vi "MultiAxisPositioningWithTime.vi"(0 "connection ID":refnum<k5>, 1 "set1":bool=TRUE, 2 "set2":bool=TRUE, 3 "set3":bool=TRUE, 4 "target1":i32, 5 "error":errorcluster, 6 "target2":i32, 7 "target3":i32) -> (14 "connection ID out":refnum<k5>, 15 "Output parameters":T1, 19 "error out":errorcluster)   [LabVIEW 2016, in "amc_api.lvlib"]
doc: "In addition to \"MultiAxisPositioning\", this function returns a timestamp to the current position of each axis."
uses:
  amc_api.lvlib
panel:
  out "jsonRespIn":string
  out "JSON-response":string="{\"jsonrpc\":\"2.0\",\"method\":\"\",\"params\":[5,1.245,true,\"name\"],\"id\":\"1\"}"
  out "JSON request":string
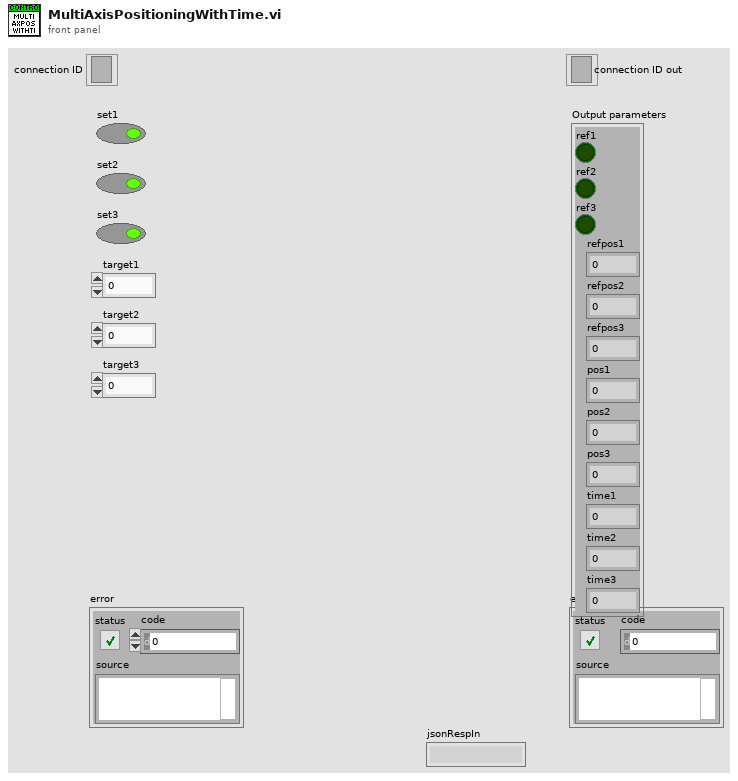
[diagram p1: front panel]
types:
  T1 = cluster{"ref1":bool, "ref2":bool, "ref3":bool, "refpos1":i32, "refpos2":i32, "refpos3":i32, "pos1":i32, "pos2":i32, "pos3":i32, "time1":dbl, "time2":dbl, "time3":dbl}
  T2 = cluster{"jsonrpc":string, "method":string, "params":string[], "id":string, "api":i32, "pid":string}
  T3 = enum16{"Standard", "Buffered", "CRLF", "Immediate"}
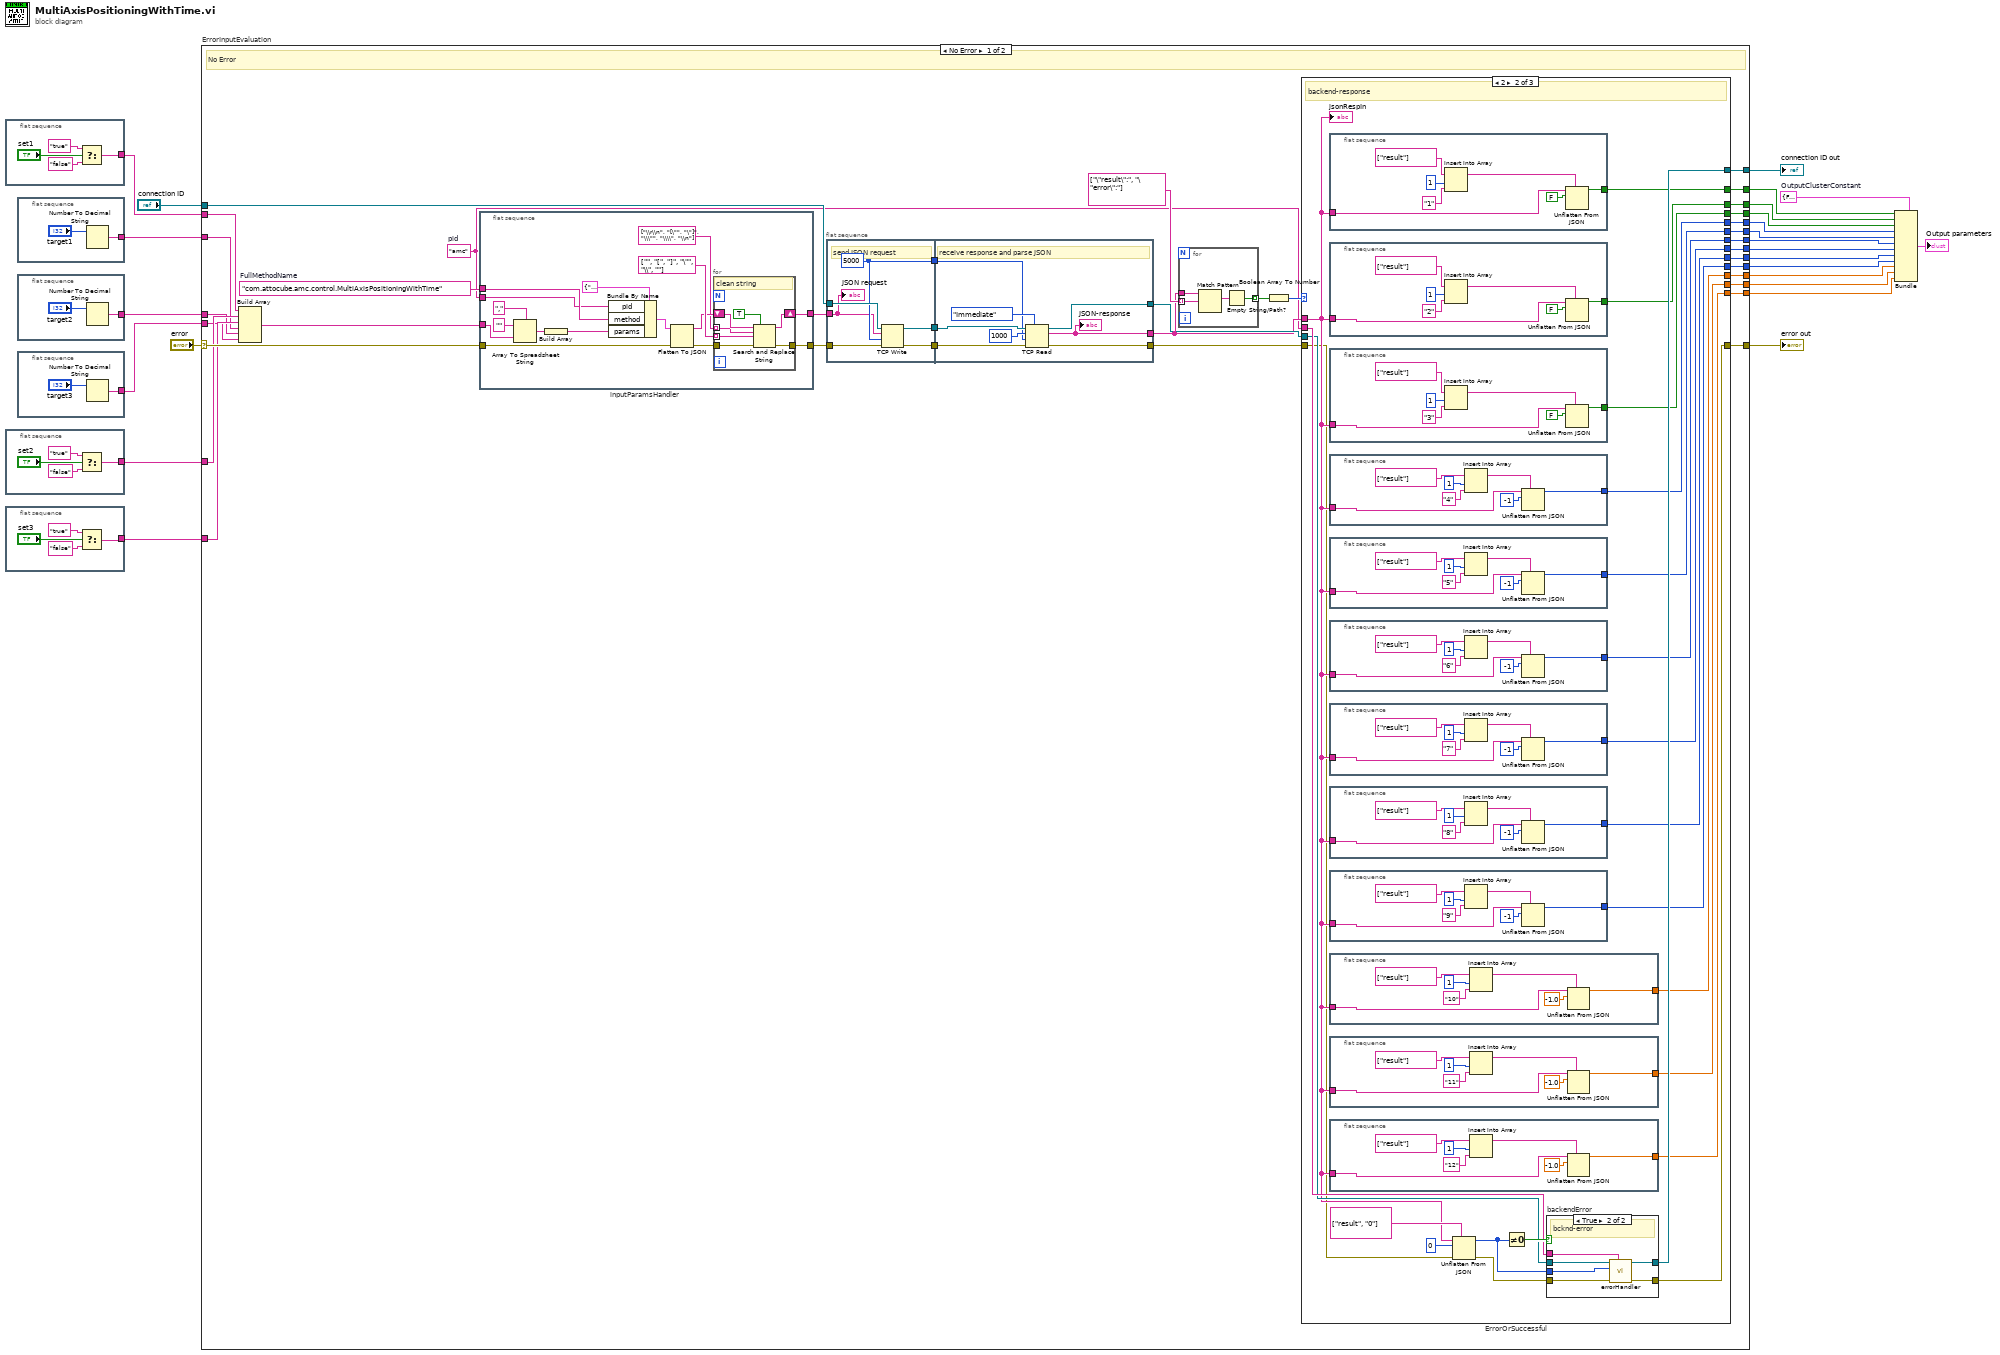
[diagram p0: block diagram]
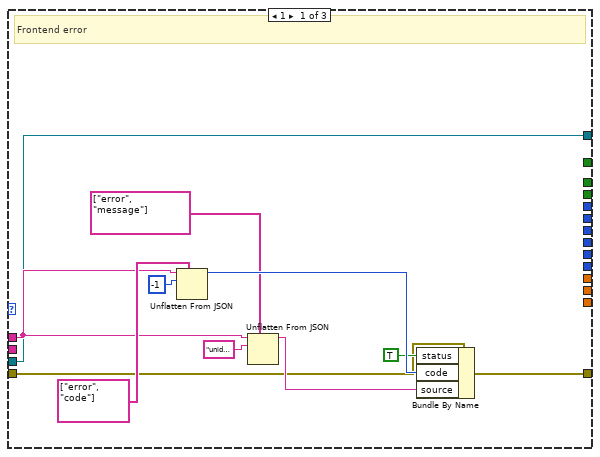
[diagram p2: hidden frame]
diagram:
  w23 = T1 {"ref1"=FALSE, "ref2"=FALSE, "ref3"=FALSE, "refpos1"=0, "refpos2"=0, "refpos3"=0, "pos1"=0, "pos2"=0, "pos3"=0, "time1"=0.0, "time2"=0.0, "time3"=0.0}  # OutputClusterConstant
  n1 = flat-sequence "in_bool" {
    tunnel: [w25] -> w19
    frame #0 {
      n2 = Select(t="true" ("Base"), s="set1", f="false" ("Base")) -> (s? t:f=w25:string)
    }
  }
  n3 = flat-sequence "in_bool" {
    tunnel: [w29] -> w18
    frame #0 {
      n4 = Select(t="true" ("Base"), s="set2", f="false" ("Base")) -> (s? t:f=w29:string)
    }
  }
  n5 = flat-sequence "in_bool" {
    tunnel: [w33] -> w17
    frame #0 {
      n6 = Select(t="true" ("Base"), s="set3", f="false" ("Base")) -> (s? t:f=w33:string)
    }
  }
  n7 = flat-sequence "in_integer" {
    tunnel: [w37] -> w16
    frame #0 {
      n8 = Number To Decimal String(number="target1") -> (decimal integer string=w37:string)  [unwired: 1 in]
    }
  }
  n9 = flat-sequence "in_integer" {
    tunnel: [w39] -> w15
    frame #0 {
      n10 = Number To Decimal String(number="target2") -> (decimal integer string=w39:string)  [unwired: 1 in]
    }
  }
  n11 = flat-sequence "in_integer" {
    tunnel: [w41] -> w14
    frame #0 {
      n12 = Number To Decimal String(number="target3") -> (decimal integer string=w41:string)  [unwired: 1 in]
    }
  }
  n13 = case "ErrorInputEvaluation" shown="No Error" "error" {
    selector: "error" -> [w71 w248]
    tunnel: "connection ID" -> [w75 w249]
    tunnel: [w62 w248] -> w22
    tunnel: [w63 w249] -> w21
    tunnel: w19 -> [w60 _]
    tunnel: w18 -> [w59 _]
    tunnel: w17 -> [w58 _]
    tunnel: w16 -> [w57 _]
    tunnel: w15 -> [w56 _]
    tunnel: w14 -> [w55 _]
    tunnel: [w54 _] -> w13
    tunnel: [w53 _] -> w12
    tunnel: [w52 _] -> w11
    tunnel: [w51 _] -> w10
    tunnel: [w50 _] -> w9
    tunnel: [w49 _] -> w8
    tunnel: [w48 _] -> w7
    tunnel: [w47 _] -> w6
    tunnel: [w46 _] -> w5
    tunnel: [w45 _] -> w4
    tunnel: [w44 _] -> w3
    tunnel: [w43 _] -> w2
    frame No Error {
      w61 = "amc"  # pid
      w72 = "com.attocube.amc.control.MultiAxisPositioningWithTime"  # FullMethodName
      # "No Error"
      n14 = Build Array ("ParametersArrayString")(w60, w59, w58, w57, w56, w55) -> (w70:string[])
      n15 = flat-sequence "inputParamsHandler" {
        tunnel: [w212] -> w69
        tunnel: w70 -> [w218]
        tunnel: w71 -> [w217]
        tunnel: [w214] -> w68
        tunnel: w72 -> [w208]
        tunnel: w61 -> [w207]
        frame #0 {
          n16 = Array To Spreadsheet String(delimiter (Tab)=",", array=w218, 3:"" ("format string")) -> (spreadsheet string=w220:string)
          n17 = Build Array "Build Array"(w220) -> (w209:string[])
          n18 = Bundle By Name(cluster=T2 {"jsonrpc"="2.0", "method"="com.attocube.amc.res.setRESReadOutFreq", "params"=[], "id"="1", "api"=2, "pid"=""} ("Cluster"), "pid"=w207, "method"=w208, "params"=w209) -> (w219:T2)
          n19 = Flatten To JSON(anything=w219, error in (no error)=w217) -> (JSON string=w213:string, 11:w215:errorcluster)  [unwired: 1 in]
          n20 = for {
            tunnel: string[] ["\\r\\n", "[\"", "\"]", "\\\"", "\\\\", "\\n"] ("search string") -> [w226] mode=indexing
            tunnel: string[] ["", "[", "]", "\"", "\\", ""] ("replace string (\"\")") -> [w225] mode=indexing
            shift-right: [w228] -> w212
            shift-left: w213 -> [w227]
            tunnel: w215 -> [w224]
            tunnel: [w223] -> w214
            # "clean string"
            n21 = Search and Replace String(replace all?=TRUE ("replace all? (F)"), input string=w227, search string=w226, replace string=w225, error in=w224) -> (result string=w228:string, error out=w223:errorcluster)  [unwired: 3 in, 2 out]
          }
        }
      }
      n22 = flat-sequence {
        tunnel: w75 -> [w239]
        tunnel: [w237] -> w78
        tunnel: [w238] -> w77
        tunnel: w68 -> [w234]
        tunnel: [w236] -> w76
        tunnel: w69 -> [w235]
        tunnel: [w243] -> w67
        tunnel: w78 -> [w245]
        tunnel: w77 -> [w244]
        tunnel: [w241] -> w66
        tunnel: w76 -> [w242]
        tunnel: [w240] -> w65
        frame #0 {
          w236 = 5000 ("timeout ms (25000)")
          # "send JSON request"
          n23 = TCP Write(connection ID=w239, data in=w235, error in (no error)=w234, 9:w236) -> (connection ID out=w237:refnum<k5>, error out=w238:errorcluster)  [unwired: 1 out]
          "JSON request" <- w235
        }
        frame #1 {
          # "receive response and parse JSON"
          n24 = TCP Read(connection ID=w245, bytes to read=1000, error in (no error)=w244, 7:T3."Immediate" ("mode (standard)"), 9:w242) -> (connection ID out=w243:refnum<k5>, data out=w240:string, error out=w241:errorcluster)
          "JSON-response" <- w240
        }
      }
      n25 = for {
        tunnel: string[] ["\"result\":", "\"error\":"] ("path") -> [w232] mode=indexing
        tunnel: [w230] -> w73 mode=indexing
        tunnel: w65 -> [w233]
        n26 = Match Pattern(string=w233, regular expression=w232) -> (match substring=w231:string)  [unwired: 1 in, 3 out]
        n27 = Empty String/Path?(string/path=w231) -> (empty?=w230:bool)
      }
      n28 = Boolean Array To Number(Boolean array=w73) -> (number=w64:u32)
      n29 = case "ErrorOrSuccessful" shown="2" w64 {
        tunnel: w65 -> [w81 w104 _]
        tunnel: w67 -> [w79 w106 w206]
        tunnel: [w79 w105 w206] -> w63
        tunnel: [w82 w102 w205] -> w62
        tunnel: w66 -> [w80 w103 w205]
        tunnel: w61 -> [_ w107 _]
        tunnel: [_ w101 _] -> w54
        tunnel: [_ w100 _] -> w53
        tunnel: [_ w99 _] -> w52
        tunnel: [_ w98 _] -> w51
        tunnel: [_ w97 _] -> w50
        tunnel: [_ w96 _] -> w49
        tunnel: [_ w95 _] -> w48
        tunnel: [_ w94 _] -> w47
        tunnel: [_ w93 _] -> w46
        tunnel: [_ w92 _] -> w45
        tunnel: [_ w91 _] -> w44
        tunnel: [_ w90 _] -> w43
        frame 1 {
          # "Frontend error"
          n30 = Unflatten From JSON(path=string[] ["error", "code"], JSON string=w81, type and defaults=-1) -> (value=w88:i32)  [unwired: 4 in, 1 out]
          n31 = Unflatten From JSON(path=string[] ["error", "message"], JSON string=w81, type and defaults="unidentified error") -> (value=w89:string)  [unwired: 4 in, 1 out]
          n32 = Bundle By Name(cluster=w80, "status"=TRUE, "code"=w88, "source"=w89) -> (w82:errorcluster)
        }
        frame 2 {
          # "backend-response"
          n33 = flat-sequence "out_bool" {
            tunnel: w104 -> [w195]
            tunnel: [w190] -> w101
            frame #0 {
              n34 = Insert Into Array "Insert Into Array"(array=string[] ["result"] ("path"), index=1, new element="1" ("idx")) -> (w192:string[])
              n35 = Unflatten From JSON(path=w192, JSON string=w195, type and defaults=FALSE) -> (value=w190:bool)  [unwired: 4 in, 1 out]
            }
          }
          n36 = flat-sequence "out_bool" {
            tunnel: w104 -> [w188]
            tunnel: [w183] -> w100
            frame #0 {
              n37 = Insert Into Array "Insert Into Array"(array=string[] ["result"] ("path"), index=1, new element="2" ("idx")) -> (w185:string[])
              n38 = Unflatten From JSON(path=w185, JSON string=w188, type and defaults=FALSE) -> (value=w183:bool)  [unwired: 4 in, 1 out]
            }
          }
          n39 = flat-sequence "out_bool" {
            tunnel: w104 -> [w181]
            tunnel: [w176] -> w99
            frame #0 {
              n40 = Insert Into Array "Insert Into Array"(array=string[] ["result"] ("path"), index=1, new element="3" ("idx")) -> (w178:string[])
              n41 = Unflatten From JSON(path=w178, JSON string=w181, type and defaults=FALSE) -> (value=w176:bool)  [unwired: 4 in, 1 out]
            }
          }
          n42 = flat-sequence "out_integer" {
            tunnel: w104 -> [w171]
            tunnel: [w169] -> w98
            frame #0 {
              n43 = Insert Into Array(array=string[] ["result"] ("path"), index=1, new element="4" ("idx")) -> (w173:string[])
              n44 = Unflatten From JSON(path=w173, JSON string=w171, type and defaults=-1 ("index")) -> (value=w169:i32)  [unwired: 4 in, 1 out]
            }
          }
          n45 = flat-sequence "out_integer" {
            tunnel: w104 -> [w164]
            tunnel: [w162] -> w97
            frame #0 {
              n46 = Insert Into Array(array=string[] ["result"] ("path"), index=1, new element="5" ("idx")) -> (w166:string[])
              n47 = Unflatten From JSON(path=w166, JSON string=w164, type and defaults=-1 ("index")) -> (value=w162:i32)  [unwired: 4 in, 1 out]
            }
          }
          n48 = flat-sequence "out_integer" {
            tunnel: w104 -> [w157]
            tunnel: [w155] -> w96
            frame #0 {
              n49 = Insert Into Array(array=string[] ["result"] ("path"), index=1, new element="6" ("idx")) -> (w159:string[])
              n50 = Unflatten From JSON(path=w159, JSON string=w157, type and defaults=-1 ("index")) -> (value=w155:i32)  [unwired: 4 in, 1 out]
            }
          }
          n51 = flat-sequence "out_integer" {
            tunnel: w104 -> [w150]
            tunnel: [w148] -> w95
            frame #0 {
              n52 = Insert Into Array(array=string[] ["result"] ("path"), index=1, new element="7" ("idx")) -> (w152:string[])
              n53 = Unflatten From JSON(path=w152, JSON string=w150, type and defaults=-1 ("index")) -> (value=w148:i32)  [unwired: 4 in, 1 out]
            }
          }
          n54 = flat-sequence "out_integer" {
            tunnel: w104 -> [w143]
            tunnel: [w141] -> w94
            frame #0 {
              n55 = Insert Into Array(array=string[] ["result"] ("path"), index=1, new element="8" ("idx")) -> (w145:string[])
              n56 = Unflatten From JSON(path=w145, JSON string=w143, type and defaults=-1 ("index")) -> (value=w141:i32)  [unwired: 4 in, 1 out]
            }
          }
          n57 = flat-sequence "out_integer" {
            tunnel: w104 -> [w136]
            tunnel: [w134] -> w93
            frame #0 {
              n58 = Insert Into Array(array=string[] ["result"] ("path"), index=1, new element="9" ("idx")) -> (w138:string[])
              n59 = Unflatten From JSON(path=w138, JSON string=w136, type and defaults=-1 ("index")) -> (value=w134:i32)  [unwired: 4 in, 1 out]
            }
          }
          n60 = flat-sequence "out_double" {
            tunnel: [w127] -> w92
            tunnel: w104 -> [w129]
            frame #0 {
              n61 = Insert Into Array(array=string[] ["result"] ("path"), index=1, new element="10" ("idx")) -> (w131:string[])
              n62 = Unflatten From JSON(path=w131, JSON string=w129, type and defaults=-1.0 ("index")) -> (value=w127:dbl)  [unwired: 4 in, 1 out]
            }
          }
          n63 = flat-sequence "out_double" {
            tunnel: [w120] -> w91
            tunnel: w104 -> [w122]
            frame #0 {
              n64 = Insert Into Array(array=string[] ["result"] ("path"), index=1, new element="11" ("idx")) -> (w124:string[])
              n65 = Unflatten From JSON(path=w124, JSON string=w122, type and defaults=-1.0 ("index")) -> (value=w120:dbl)  [unwired: 4 in, 1 out]
            }
          }
          n66 = flat-sequence "out_double" {
            tunnel: [w113] -> w90
            tunnel: w104 -> [w115]
            frame #0 {
              n67 = Insert Into Array(array=string[] ["result"] ("path"), index=1, new element="12" ("idx")) -> (w117:string[])
              n68 = Unflatten From JSON(path=w117, JSON string=w115, type and defaults=-1.0 ("index")) -> (value=w113:dbl)  [unwired: 4 in, 1 out]
            }
          }
          n69 = Unflatten From JSON(path=string[] ["result", "0"], JSON string=w104, type and defaults=0, error in (no error)=w103) -> (value=w108:i32, error out=w110:errorcluster)  [unwired: 3 in]
          n70 = Not Equal To 0?(x=w108) -> (x != 0?=w109:bool)
          n71 = case "backendError" shown="True" w109 {
            tunnel: w108 -> [_ w204]
            tunnel: w110 -> [w198 w203]
            tunnel: [w197 w202] -> w105
            tunnel: [w198 w201] -> w102
            tunnel: w106 -> [w197 w200]
            tunnel: w107 -> [_ w199]
            frame False {
              # "successful"
            }
            frame True {
              # "bcknd-error"
              n72 = call "errorHandler.vi"("pid"=w199, "error in"=w203, "errNbr"=w204, "connection ID"=w200) -> ("error out 2"=w201:errorcluster, "connection ID out"=w202:refnum<k5>)  [unwired: 6 in]
            }
          }
          "jsonRespIn" <- w104
        }
        frame Default {
          # "NoResponse"
        }
      }
    }
    frame Error {
      # "Error"
    }
  }
  "error out" <- w22
  "connection ID out" <- w21
  n73 = Bundle ("BundleOutputs")(cluster=w23, "ref1"=w13, "ref2"=w12, "ref3"=w11, "refpos1"=w10, "refpos2"=w9, "refpos3"=w8, "pos1"=w7, "pos2"=w6, "pos3"=w5, "time1"=w4, "time2"=w3, "time3"=w2) -> (→"Output parameters":T1)
